vi "Try_Updating_Files.vi"() -> ()   [LabVIEW 2022 SP3]
uses:
  Globals/Constants_global.vi
panel:
  out "Files to update":string[][](array[string])
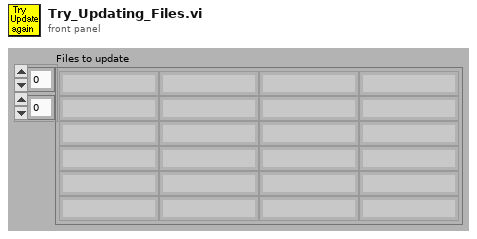
[diagram p1: front panel]
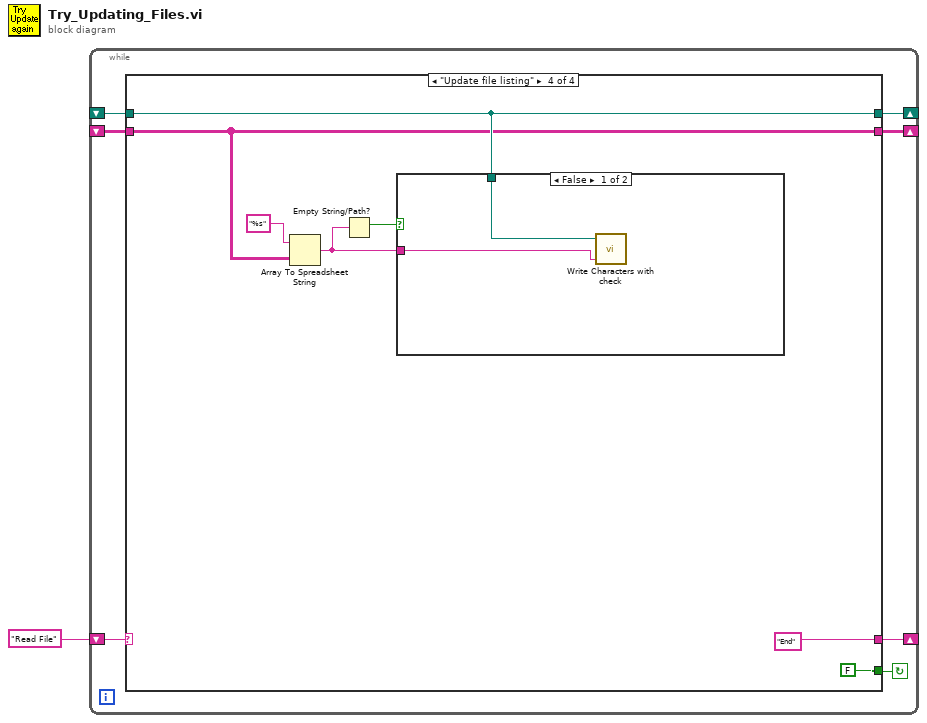
[diagram p0: block diagram]
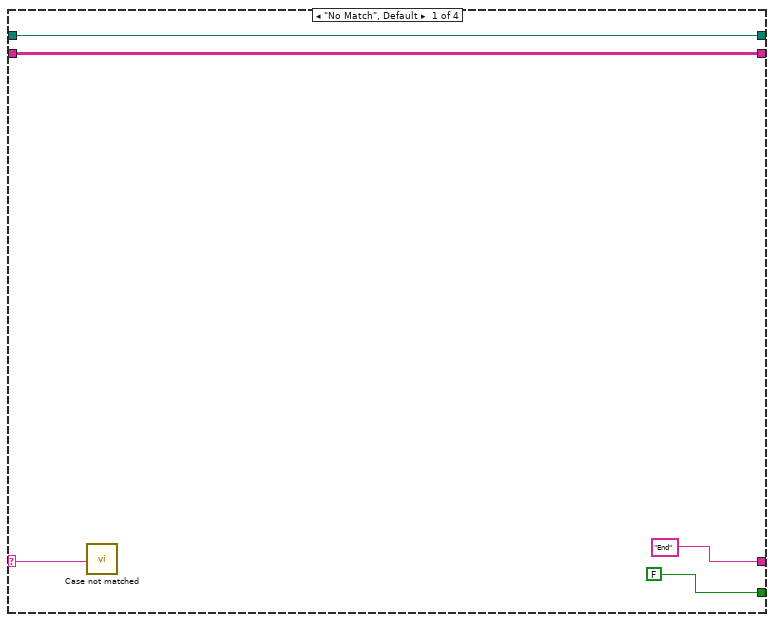
[diagram p2: hidden frame]
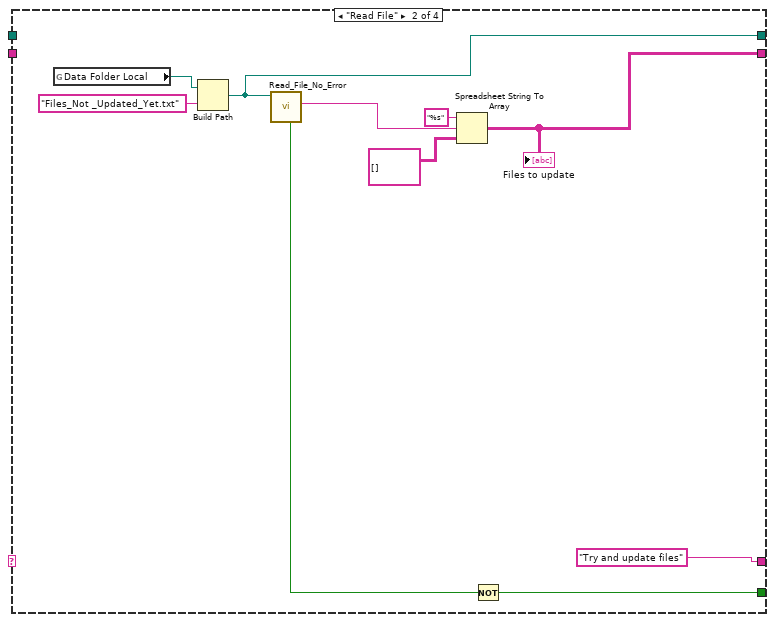
[diagram p3: hidden frame]
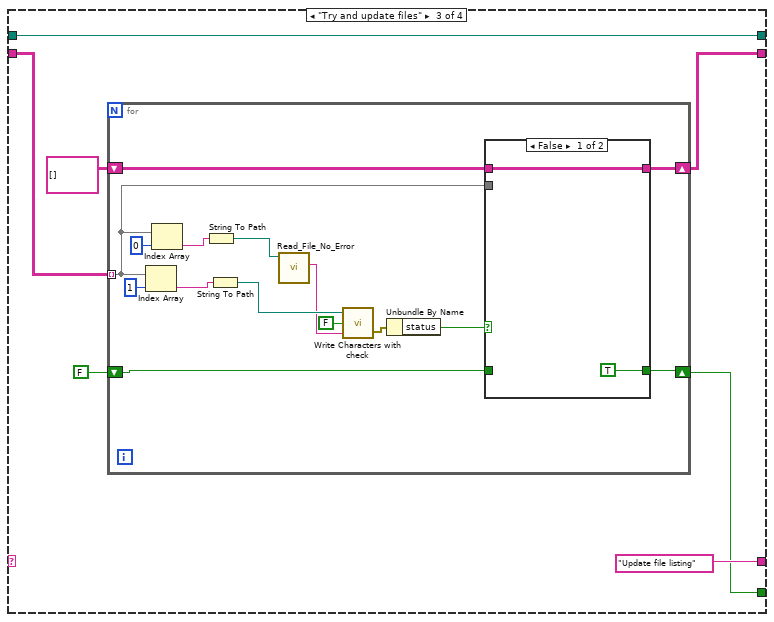
[diagram p4: hidden frame]
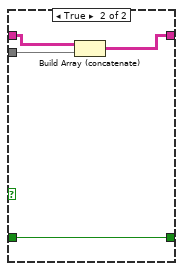
[diagram p5: hidden frame]
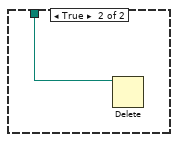
[diagram p6: hidden frame]
diagram:
  n1 = while {
    shift-left: "Read File" -> [w6]
    shift-right: [w7] -> _
    shift-right: [w5] -> _
    shift-left: _ -> [w3]
    shift-right: [w4] -> _
    shift-left: _ -> [w2]
    stop <- w8 continue-if-true
    n2 = case shown="\"Update file listing\"" w6 {
      selector: w6 -> [w9 _ _ _]
      tunnel: [FALSE w19 w25 FALSE ("status")] -> w8
      tunnel: ["End" "Try and update files" "Update file listing" "End"] -> w7
      tunnel: [w11 w21 w29 w57] -> w5
      tunnel: [w10 w16 w27 w55] -> w4
      tunnel: w3 -> [w11 _ w29 w57]
      tunnel: w2 -> [w10 _ w26 w55]
      frame "No Match", Default {
        n3 = call "Case not matched.vi"("Case Name not Matched"=w9) -> ()
      }
      frame "Read File" {
        n4 = global read "Constants_global.vi" "Data Folder Local"() -> (w23:path)
        n5 = Build Path(base path=w23, name or relative path="Files_Not _Updated_Yet.txt") -> (appended path=w21:path)
        n6 = call "Read_File_No_Error.vi"("Filename"=w21) -> ("Error?"=w20:bool, "string"=w18:string)  [unwired: 2 in, 6 out]
        n7 = Spreadsheet String To Array(format string="%s", spreadsheet string=w18, array type (2D Dbl)=string[][] []) -> (array=w16:string[][])  [unwired: 1 out]
        "Files to update" <- w16
        n8 = Not(x=w20) -> (.not. x?=w19:bool)
      }
      frame "Try and update files" {
        n9 = for {
          tunnel: w26 -> [w39] mode=indexing
          shift-right: [w37] -> w27
          shift-left: string[][] [] -> [w38]
          shift-right: [w36] -> w25
          shift-left: FALSE -> [w35]
          n10 = Index Array(array=w39, index=1) -> (element=w42:string)
          n11 = Index Array(array=w39, index=0) -> (element=w43:string)
          n12 = String To Path(string=w43) -> (path=w41:path)
          n13 = String To Path(string=w42) -> (path=w34:path)
          n14 = call "Read_File_No_Error.vi"("Filename"=w41) -> ("string"=w33:string)  [unwired: 2 in, 7 out]
          n15 = call "Write Characters with check.vi"("String to Write"=w33, "Call EnFlo Error Handler?"=FALSE, "file (use dialog)"=w34) -> ("error out"=w31:errorcluster)  [unwired: 1 in]
          n16 = Unbundle By Name(w31) -> ("status"=w40:bool)
          n17 = case shown="False" w40 {
            tunnel: w39 -> [_ w51]
            tunnel: w38 -> [w47 w50]
            tunnel: [w47 w49] -> w37
            tunnel: [TRUE w48] -> w36
            tunnel: w35 -> [_ w48]
            frame False {
            }
            frame True {
              n18 = Build Array (concatenate)(w50, w51) -> (w49:string[][])
            }
          }
        }
      }
      frame "Update file listing" {
        n19 = Array To Spreadsheet String(array=w55, 3:"%s" ("format string")) -> (spreadsheet string=w53:string)  [unwired: 1 out]
        n20 = Empty String/Path?(string/path=w53) -> (empty?=w52:bool)
        n21 = case shown="False" w52 {
          tunnel: w57 -> [w60 w61]
          tunnel: w53 -> [w59 _]
          frame False {
            n22 = call "Write Characters with check.vi"("String to Write"=w59, "file (use dialog)"=w60) -> ()  [unwired: 2 in, 1 out]
          }
          frame True {
            n23 = Delete(path (use dialog)=w61) -> ()  [unwired: 1 in, 6 out]
          }
        }
      }
    }
  }
